vi "Test Set PSU.vi"(6 "Axis":T1=enum."Z", 8 "error in (no error)":errorcluster, 11 "Instrument.OxfordVRM in":refnum<class "Instrument.OxfordVRM.lvclass">) -> (0 "error out":errorcluster, 3 "Instrument.OxfordVRM out":refnum<class "Instrument.OxfordVRM.lvclass">)   [LabVIEW 2019, in "Instrument.OxfordVRM.lvclass"]
uses:
  Instrument.OxfordVRM.lvclass
  <vilib>/addons/_JKI Toolkits/Caraya/classes/Test/Test.lvclass
  <vilib>/addons/_JKI Toolkits/Caraya/classes/Assert/Assert.lvclass
  <vilib>/addons/_JKI Toolkits/Caraya/classes/Assert/Assert Not Error.vi
  <vilib>/addons/_JKI Toolkits/Caraya/classes/Assert/Assert Equal Value and Type_Variant.vi
  <userlib>/LevyLab/Instrument Framework/Instrument Types/Cryostat/Typedefs/Magnet Axis--Enum.ctl
  <userlib>/LevyLab/Instrument Framework/Instrument Types/Cryostat/Instrument.Cryostat.lvclass
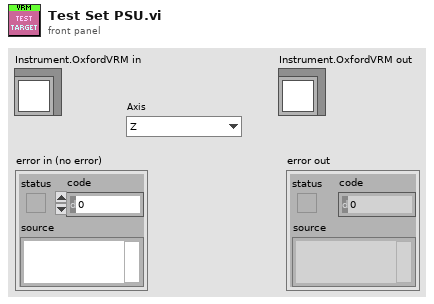
[diagram p1: front panel]
types:
  T1 = typedef "Instrument.Cryostat.lvclass/Magnet Axis--Enum.ctl" = enum16{"X", "Y", "Z"}
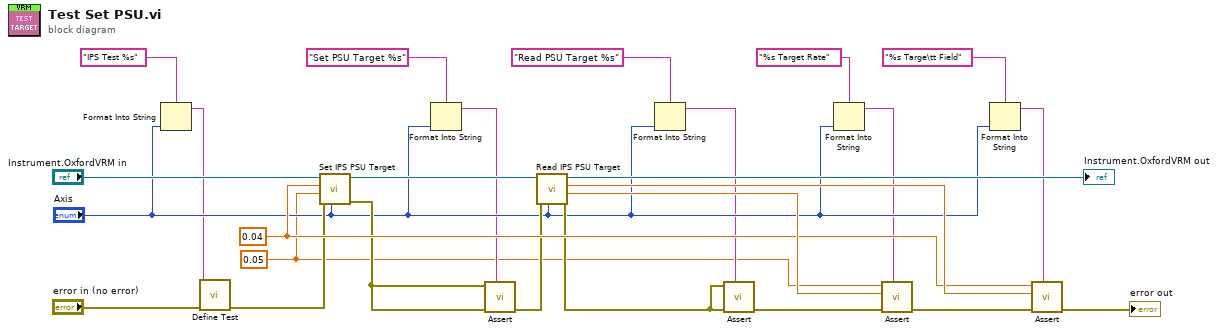
[diagram p0: block diagram]
diagram:
  w1 = 0.05 ("Target Field Rate (T/min)")
  w19 = 0.04 ("Target Field (T)")
  n1 = Format Into String(format string="IPS Test %s" ("Label (VI Title)"), "Axis") -> (resulting string=w2:string)  [unwired: 2 in, 1 out]
  n2 = call <vilib>:"Define Test.vi"("error in (no error)"="error in (no error)", "Label (VI Title)"=w2) -> ("error out"=w14:errorcluster)  [unwired: 8 in, 1 out]
  n3 = call "Set IPS PSU Target.vi"("Axis"="Axis", "error in (no error)"=w14, "Target Field Rate (T/min)"=w1, "Target Field (T)"=w19, "Instrument.OxfordVRM in"="Instrument.OxfordVRM in") -> ("error out"=w15:errorcluster, "Instrument.OxfordVRM out"=w18:refnum<class "Instrument.OxfordVRM.lvclass">)  [unwired: 4 in, 1 out]
  n4 = Format Into String(format string="Set PSU Target %s" ("Label"), "Axis") -> (resulting string=w5:string)  [unwired: 2 in, 1 out]
  n5 = call-poly <vilib>:"Assert.vi"("Label"=w5, "error in (no error)"=w15, "Not Error?"=w15) -> ("error out"=w16:errorcluster)  [unwired: 7 in, 1 out]
  n6 = call "Read IPS PSU Target.vi"("Axis"="Axis", "error in (no error)"=w16, "Instrument.OxfordVRM in"=w18) -> ("error out"=w13:errorcluster, "Target Field Rate (T/min)"=w24:dbl, "Target Field (T)"=w23:dbl, "Instrument.OxfordVRM out"=→"Instrument.OxfordVRM out":refnum<class "Instrument.OxfordVRM.lvclass">)  [unwired: 5 in]
  n7 = Format Into String(format string="Read PSU Target %s" ("Label"), "Axis") -> (resulting string=w6:string)  [unwired: 2 in, 1 out]
  n8 = call-poly <vilib>:"Assert.vi"("Label"=w6, "error in (no error)"=w13, "Not Error?"=w13) -> ("error out"=w26:errorcluster)  [unwired: 7 in, 1 out]
  n9 = Format Into String(format string="%s Target Rate" ("Label"), "Axis") -> (resulting string=w4:string)  [unwired: 2 in, 1 out]
  n10 = call-poly <vilib>:"Assert.vi"("Label"=w4, "error in (no error)"=w26, "Y"=w24, "X"=w1) -> ("error out"=w25:errorcluster)  [unwired: 6 in, 1 out]
  n11 = Format Into String(format string="%s Targe\tt Field" ("Label"), "Axis") -> (resulting string=w3:string)  [unwired: 2 in, 1 out]
  n12 = call-poly <vilib>:"Assert.vi"("Label"=w3, "error in (no error)"=w25, "Y"=w23, "X"=w19) -> ("error out"=→"error out":errorcluster)  [unwired: 6 in, 1 out]
